vi "Test Mode Pcb Comp Optimize.vi"(6 "PcbComp21Offs":i32, 7 "PcbComp20Offs":i32, 8 "error in (no error)":errorcluster caption="错误输入（无错误）", 9 "PcbComp10Offs":i32, 10 "PcbAttOffs":i32, 11 "asicHandle":i32) -> (0 "error out":errorcluster caption="错误输出", 3 "function return":i32)   [LabVIEW 2018]
doc: "extern int __stdcall APSxTestModePcbCompOptimize (int asicHandle, IN int PcbAttOffs, IN int PcbComp10Offs, IN int PcbComp20Offs, IN int PcbComp21Offs);"
uses:
  APSx.dll/APSx.dll
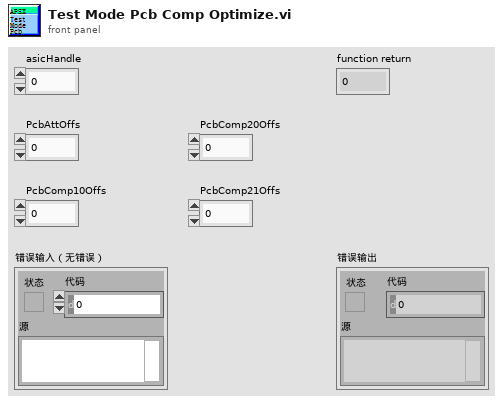
[diagram p1: front panel]
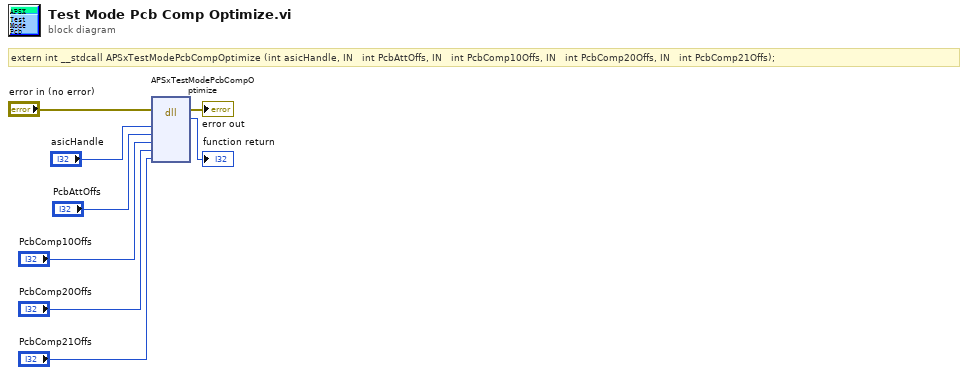
[diagram p0: block diagram]
diagram:
  # "extern int __stdcall APSxTestModePcbCompOptimize (int asicHandle, IN   int PcbAttOffs, IN   int PcbComp10Offs, IN   int PcbComp20Offs, IN   int PcbComp21Offs);"
  n1 = dll-call lib="PTH2[abs D项目Feng恒隆项目Labview传感器对中台SourcesAPSx.dllAPSx.*" fn="APSxTestModePcbCompOptimize"(error in="error in (no error)", "asicHandle"="asicHandle", "PcbAttOffs"="PcbAttOffs", "PcbComp10Offs"="PcbComp10Offs", "PcbComp20Offs"="PcbComp20Offs", "PcbComp21Offs"="PcbComp21Offs") -> (error out=→"error out":errorcluster, →"function return":i32)  [unwired: 7 in, 1 out]
